vi "light_grid.vi"(9 "Array":bool[](array[boolean]), 11 "Boolean":bool=TRUE) -> (1 "Array 2":bool[](array[boolean]), 3 "logical AND":bool)   [LabVIEW 2017]
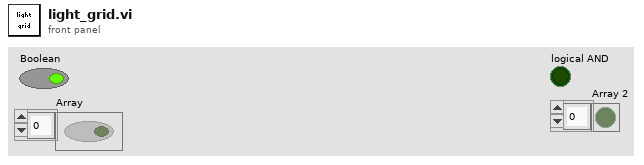
[diagram p1: front panel]
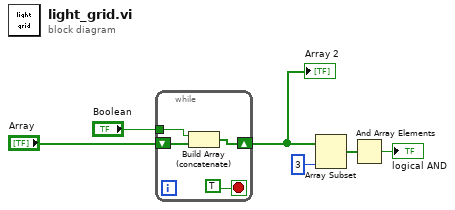
[diagram p0: block diagram]
diagram:
  n1 = while {
    tunnel: "Boolean" -> [w9]
    shift-right: [w8] -> w4
    shift-left: "Array" -> [w7]
    stop <- TRUE stop-if-true
    n2 = Build Array (concatenate)(w9, w7) -> (w8:bool[])
  }
  "Array 2" <- w4
  n3 = Array Subset ("数组子集")(array=w4, length=3) -> (w5:bool[])  [unwired: 1 in]
  n4 = And Array Elements(Boolean array=w5) -> (logical AND=→"logical AND":bool)
